vi "double array insert.vi"(0 "Element":dbl, 2 "Array in":dbl[](array[numeric]), 5 "Index":i32) -> (3 "Array size":dbl, 4 "Array out":dbl[](array[numeric]))   [LabVIEW 2014]
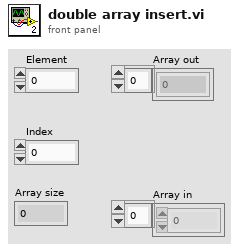
[diagram p1: front panel]
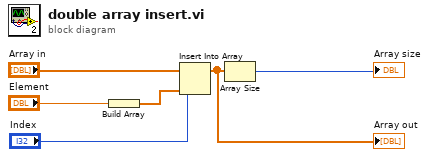
[diagram p0: block diagram]
diagram:
  n1 = Build Array("Element") -> (w5:dbl[])
  n2 = Insert Into Array(array="Array in", index="Index", new element=w5) -> (w6:dbl[])
  "Array out" <- w6
  n3 = Array Size(array=w6) -> (size(s)=→"Array size":i32)
